vi "GEA2 Serial Command Length.vi"(6 "Current Read Index":i32, 8 "Error In":errorcluster, 9 "CRCArray":u8[](array[numeric]), 10 "ReadArray":u8[](array[numeric]), 11 "Total Bytes Read":i32) -> (0 "Error Out":errorcluster, 1 "Bytes Remaining":u8, 2 "CRC Array":u8[](array[numeric]), 3 "Current Read Index":i32, 4 "Boolean":bool, 5 "Length":u8)   [LabVIEW 2014]
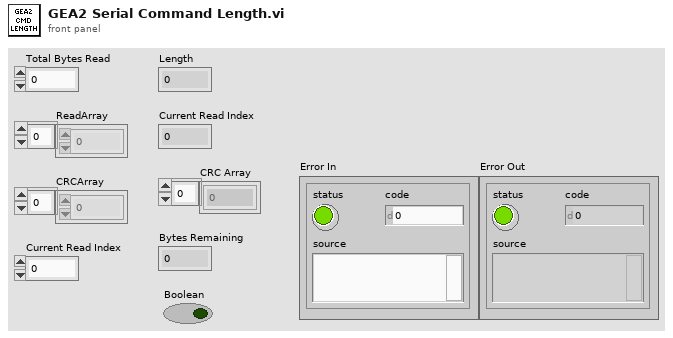
[diagram p1: front panel]
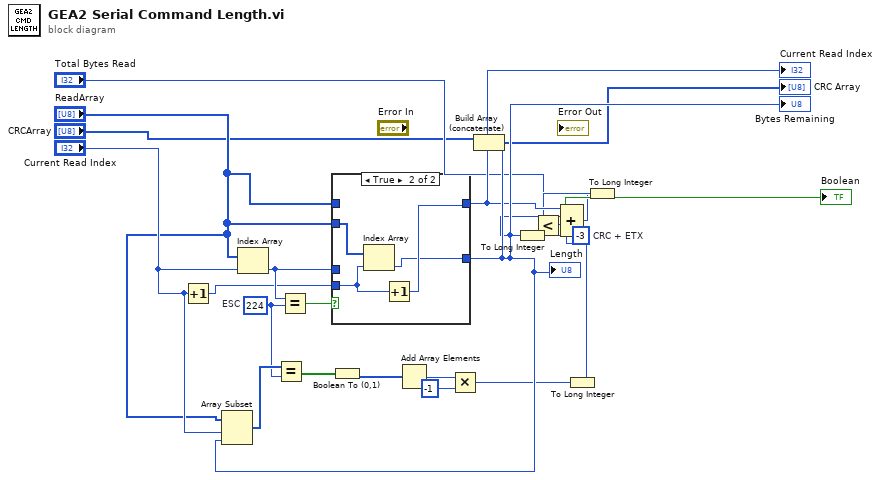
[diagram p0: block diagram]
diagram:
  w4 = -3  # CRC + ETX
  w13 = u8 224  # ESC
  n1 = Increment(x="Current Read Index") -> (x+1=w7:i32)
  n2 = Index Array(array="ReadArray", index="Current Read Index") -> (element=w8:u8)
  n3 = Equal?(x=w8, y=w13) -> (x = y?=w1:bool)
  n4 = case shown="True" w1 {
    tunnel: [w24 w26] -> w22
    tunnel: [w25 w27] -> w11
    tunnel: "ReadArray" -> [_ _]
    tunnel: "ReadArray" -> [_ w29]
    tunnel: w7 -> [w25 w28]
    tunnel: w8 -> [w24 _]
    frame False {
    }
    frame True {
      n5 = Index Array(array=w29, index=w28) -> (element=w26:u8)
      n6 = Increment(x=w28) -> (x+1=w27:i32)
    }
  }
  "Length" <- w22
  "Bytes Remaining" <- w22
  "Current Read Index" <- w11
  n7 = Array Subset(array="ReadArray", index="Current Read Index", length=w22) -> (w23:u8[])
  n8 = Equal?(x=w23, y=w13) -> (x = y?=w14:bool[])
  n9 = Boolean To (0,1)(Boolean=w14) -> (0, 1=w15:i16[])
  n10 = Add Array Elements(numeric array=w15) -> (sum=w16:i16)
  n11 = Multiply(x=w16, y=i16 -1) -> (x*y=w18:i16)
  n12 = Build Array (concatenate)("CRCArray", w22) -> (→"CRC Array":u8[])
  n13 = To Long Integer(number=w22) -> (32bit integer=w12:i32)
  n14 = To Long Integer(number=w18) -> (32bit integer=w19:i32)
  n15 = Compound Arithmetic op=ADD(w11, w4, w12, w19) -> (w5:i32)
  n16 = To Long Integer(number=w5) -> (32bit integer=w10:i32)
  n17 = Less?(x="Total Bytes Read", y=w10) -> (x < y?=→"Boolean":bool)
